vi "Interface 1.vi"() -> ()   [LabVIEW 2013]
panel:
  in  "stop":bool
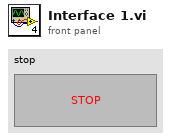
[diagram p1: front panel]
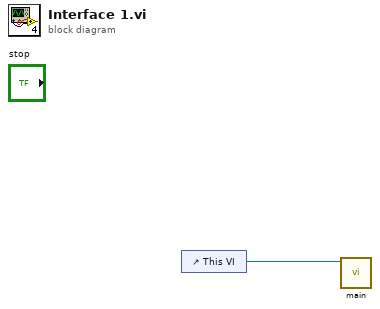
[diagram p0: block diagram]
diagram:
  n1 = control-ref of="This VI"() -> (w1:refnum<vi>)
  n2 = call "main.vi"("VI Refnum"=w1) -> ()  [unwired: 11 in]
